vi "WT300 Get Power.vi"(8 "error in (no error)":errorcluster, 10 "Update Rate (500m s)":dbl(ring)=0.5 format="%#_2f" items=["100m"=0.1, "250m"=0.25, "500m"=0.5, "1"=1.0, "2"=2.0, "5"=5.0], 11 "VISA Refnum in":refnum<visa-resource-name>) -> (0 "error out":errorcluster, 1 "Function":string[](array[string]), 2 "Measurement":dbl[](array[numeric]), 3 "VISA Refnum out":refnum<visa-resource-name>)   [LabVIEW 2019]
uses:
  Public/Utility/Function/Create Function String (Power).vi
  Public/Data/Read Measurement (Normal).vi
  Yokogawa WT300 Series.lvlib
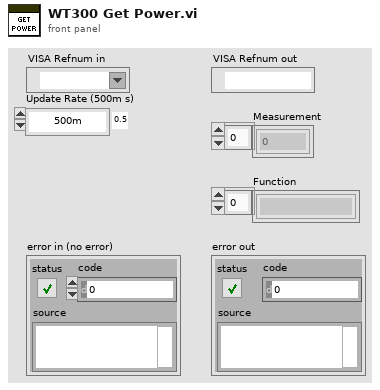
[diagram p1: front panel]
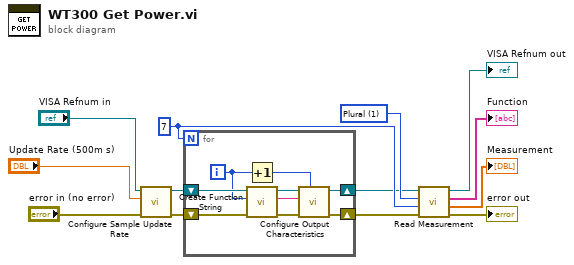
[diagram p0: block diagram]
diagram:
  w13 = 7
  w8 = 1 items=["One", "Plural"] ("Measure Item (1: Plural)")
  n1 = call "Configure Sample Update Rate.vi"("error in (no error)"="error in (no error)", "Update Rate (500m s)"="Update Rate (500m s)", "VISA resource name"="VISA Refnum in") -> ("error out"=w4:errorcluster, "VISA resource name out"=w3:refnum<visa-resource-name>)  [unwired: 7 in]
  n2 = for {
    N: w13 -> [_]
    shift-right: [w16] -> w7
    shift-left: w3 -> [w22]
    shift-right: [w17] -> w6
    shift-left: w4 -> [w21]
    i -> [w15]
    n3 = Increment(x=w15) -> (x+1=w14:i32)
    n4 = call-poly "Create Function String.vi"("error in (no error)"=w21, "Function (0: P)"=w15, "VISA resource name"=w22) -> ("error out"=w18:errorcluster, "Function String"=w20:string, "VISA resource name out"=w19:refnum<visa-resource-name>)  [unwired: 6 in]
    n5 = call "Configure Output Characteristics.vi"("Item (1)"=w14, "error in (no error)"=w18, "Function (Empty)"=w20, "VISA resource name"=w19) -> ("error out"=w17:errorcluster, "VISA resource name out"=w16:refnum<visa-resource-name>)  [unwired: 6 in]
  }
  n6 = call-poly "Read Measurement.vi"("error in (no error)"=w6, "Number of Item (15)"=w13, "Measure Item (1: Plural)"=w8, "VISA resource name"=w7) -> ("error out"=→"error out":errorcluster, "Measurement"=→"Measurement":dbl[], "Function"=→"Function":string[], "VISA resource name out"=→"VISA Refnum out":refnum<visa-resource-name>)  [unwired: 4 in]
